vi "ChangeToStaveCoordinateFrame (SubVI).vi"(0 "Loaded array (image frame)":dbl[][](array[numeric]), 1 "Image Origin in XYZ Stage Coords [mm]":dbl[](array[numeric]), 2 "Units":T1(ring), 3 "Pixel resolution":dbl=3.5) -> (5 "Array (stage frame, mm)":dbl[][](array[numeric]))   [LabVIEW 2016]
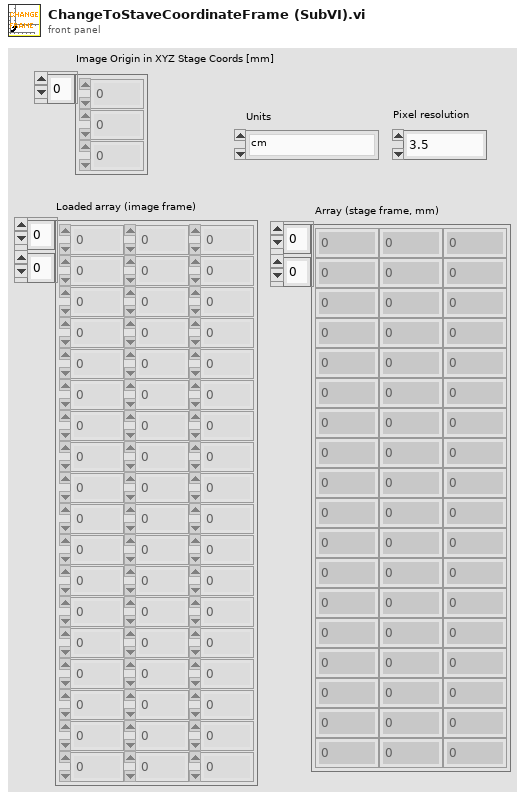
[diagram p1: front panel]
types:
  T1 = enum16{"cm", "mm", "pixels [mm/pix]", "pixels [um/pix]"}
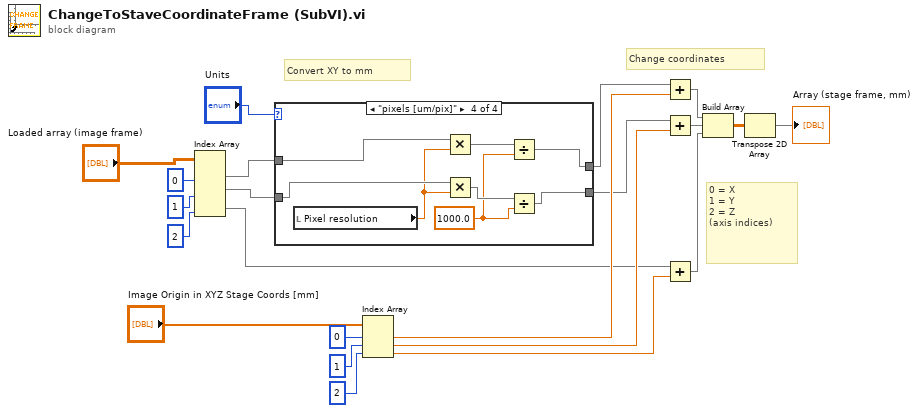
[diagram p0: block diagram]
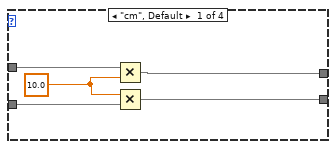
[diagram p2: hidden frame]
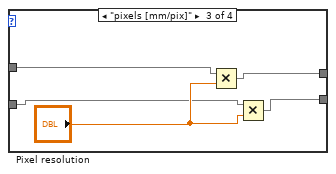
[diagram p4: hidden frame]
diagram:
  # "Convert XY to mm"
  # "Change coordinates"
  # "0 = X\n1 = Y\n2 = Z\n(axis indices)"
  n1 = Index Array(array="Loaded array (image frame)", index (col) #1=0 ("index (row)"), index (col) #2=1 ("index (row)"), index (col) #3=2 ("index (row)")) -> (element #1=w9:dbl[], element #2=w8:dbl[], element #3=w5:dbl[])  [unwired: 3 in]
  n2 = case shown="\"pixels [um/pix]\"" "Units" {
    tunnel: [w24 w29 w30 w40] -> w7
    tunnel: w9 -> [w27 w29 w31 w41]
    tunnel: w8 -> [w25 w28 w33 w39]
    tunnel: [w23 w28 w32 w35] -> w6
    frame "cm", Default {
      w26 = 10.0 ("y")
      n3 = Multiply(x=w27, y=w26) -> (x*y=w24:dbl[])
      n4 = Multiply(x=w26, y=w25) -> (x*y=w23:dbl[])
    }
    frame "mm" {
    }
    frame "pixels [mm/pix]" {
      n5 = Multiply(x=w31, y="Pixel resolution") -> (x*y=w30:dbl[])
      n6 = Multiply(x=w33, y="Pixel resolution") -> (x*y=w32:dbl[])
    }
    frame "pixels [um/pix]" {
      w36 = 1000.0
      n7 = local read "Pixel resolution"() -> (w38:dbl)
      n8 = Multiply(x=w41, y=w38) -> (x*y=w42:dbl[])
      n9 = Multiply(x=w39, y=w38) -> (x*y=w37:dbl[])
      n10 = Divide(x=w42, y=w36) -> (x/y=w40:dbl[])
      n11 = Divide(x=w37, y=w36) -> (x/y=w35:dbl[])
    }
  }
  n12 = Index Array(array="Image Origin in XYZ Stage Coords [mm]", index #1=0 ("index"), index #2=1 ("index (row)"), index #3=2 ("index (row)")) -> (element #1=w18:dbl, element #2=w14:dbl, element #3=w13:dbl)
  n13 = Add(x=w7, y=w18) -> (x+y=w12:dbl[])
  n14 = Add(x=w6, y=w14) -> (x+y=w11:dbl[])
  n15 = Add(x=w5, y=w13) -> (x+y=w10:dbl[])
  n16 = Build Array(w12, w11, w10) -> (w3:dbl[][])
  n17 = Transpose 2D Array(2D array=w3) -> (transposed array=→"Array (stage frame, mm)":dbl[][])
